vi "table path.vi"(8 "error in":errorcluster, 11 "Data Form":T1={"Dimensions"={"Dim X"=0, "Dim Y"=0, "Dim Z"=0}, "Folder XRF Files"=path "", "Dynamic Load"=FALSE, "Data From Vitruvio?"=TRUE}) -> (0 "error out":errorcluster, 3 "path tables":path)   [LabVIEW 2023]
uses:
  control/Data Form.ctl
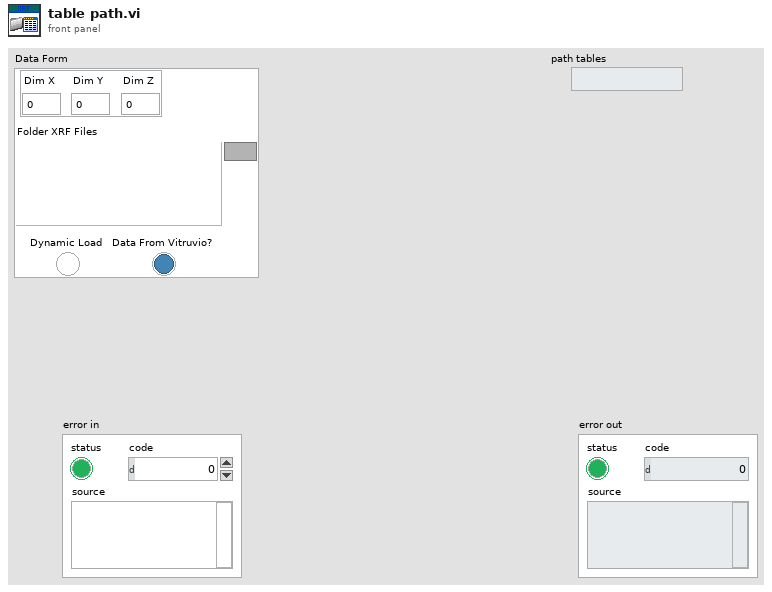
[diagram p1: front panel]
types:
  T1 = typedef "Data Form.ctl" = cluster{"Dimensions":cluster{"Dim X":i32, "Dim Y":i32, "Dim Z":i32}, "Folder XRF Files":path, "Dynamic Load":bool, "Data From Vitruvio?":bool}
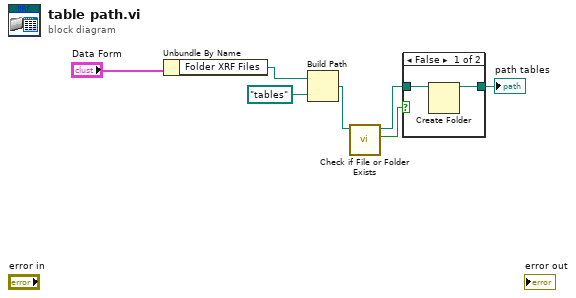
[diagram p0: block diagram]
diagram:
  n1 = Unbundle By Name("Data Form") -> ("Folder XRF Files"=w3:path)
  n2 = Build Path(base path=w3, name or relative path=path "tables") -> (appended path=w4:path)
  n3 = call <vilib>:"Check if File or Folder Exists.vi"("path"=w4) -> ("file or folder exists?"=w6:bool, "dup path"=w5:path)  [unwired: 8 in, 1 out]
  n4 = case shown="False" w6 {
    tunnel: w5 -> [w9 w10]
    tunnel: [w8 w10] -> w2
    frame False {
      n5 = Create Folder(path (use dialog)=w9) -> (created path=w8:path)  [unwired: 2 in, 2 out]
    }
    frame True {
    }
  }
  "path tables" <- w2
